vi "Get Data In Terminal.vi"(8 "error in (no error)":errorcluster, 11 "Terms[]":refnum<vi>[](array[refnum])) -> (0 "error out":errorcluster, 2 "Terminal out":refnum<vi>)   [LabVIEW 2018]
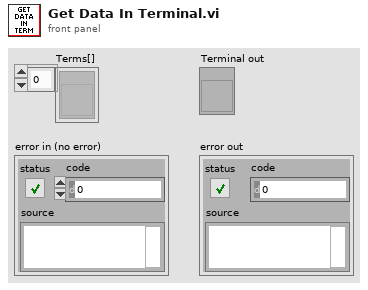
[diagram p1: front panel]
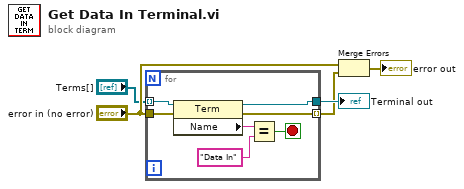
[diagram p0: block diagram]
diagram:
  n1 = for {
    tunnel: [w12] -> w5
    tunnel: [w11] -> w1 mode=indexing
    tunnel: "Terms[]" -> [w10] mode=indexing
    tunnel: "error in (no error)" -> [w9]
    stop <- w6 stop-if-true
    n2 = property class="Term"(reference=w10, error in=w9) -> (reference out=w12:refnum<vi>, error out=w11:errorcluster, "Name"=w7:string)
    n3 = Equal?(x=w7, y="Data In") -> (x = y?=w6:bool)
  }
  "Terminal out" <- w5
  n4 = Merge Errors("error in (no error)", w1) -> (→"error out":errorcluster)
